vi "Select TCP Queue.vi"(8 "error in (no error)":errorcluster, 11 "DAQ Actor in":refnum<class "DAQ Actor.lvclass">) -> (0 "error out":errorcluster, 2 "TCP Queue":refnum<class "Message Enqueuer.lvclass">, 3 "DAQ Actor out":refnum<class "DAQ Actor.lvclass">)   [LabVIEW 2018, in "Data Acquisition.lvlib" / "DAQ Actor.lvclass"]
uses:
  DAQ Actor.lvclass
  <vilib>/ActorFramework/Message Enqueuer/Message Enqueuer.lvclass
  DAQ Actor.lvclass/DAQ Actor.ctl
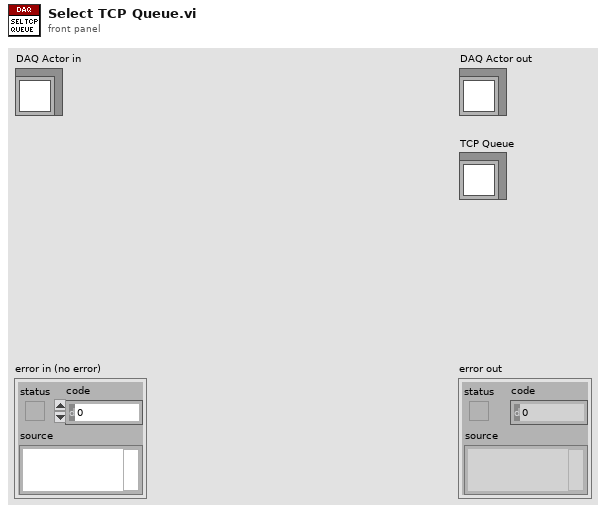
[diagram p1: front panel]
types:
  T1 = typedef "TE_Designator.ctl" = enum16{"High Speed", "Low Speed"}
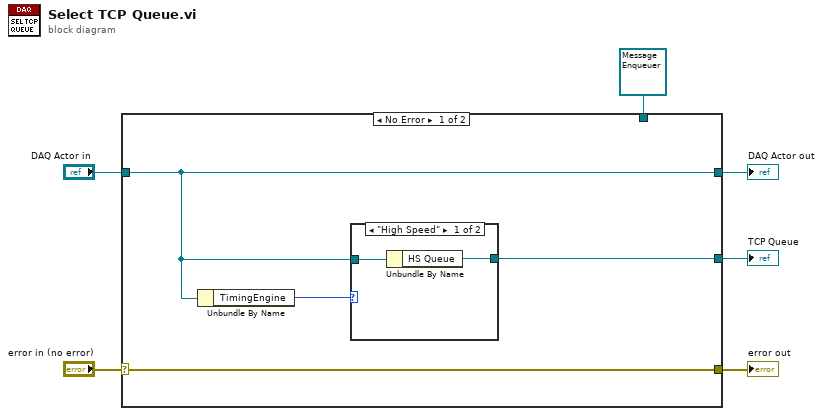
[diagram p0: block diagram]
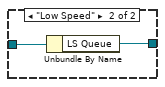
[diagram p2: hidden frame]
diagram:
  n1 = case shown="No Error" "error in (no error)" {
    selector: "error in (no error)" -> [w7 w17]
    tunnel: [w7 w17] -> w5
    tunnel: [w10 w16] -> w3
    tunnel: "DAQ Actor in" -> [w10 w16]
    tunnel: [w9 w15] -> w2
    tunnel: refnum<class "Message Enqueuer.lvclass"> refnum ("LS Queue") -> [_ w15]
    frame No Error {
      n2 = Unbundle By Name(w10) -> ("TimingEngine"=w8:T1)
      n3 = case shown="\"High Speed\"" w8 {
        tunnel: w10 -> [w12 w14]
        tunnel: [w11 w13] -> w9
        frame "High Speed" {
          n4 = Unbundle By Name(w12) -> ("HS Queue"=w11:refnum<class "Message Enqueuer.lvclass">)
        }
        frame "Low Speed" {
          n5 = Unbundle By Name(w14) -> ("LS Queue"=w13:refnum<class "Message Enqueuer.lvclass">)
        }
      }
    }
    frame Error {
    }
  }
  "error out" <- w5
  "DAQ Actor out" <- w3
  "TCP Queue" <- w2
